vi "setIDtoVD.vi"(0 "Interface in":T4, 5 "IDtoVD":T1={"gains"={"proportional gain"=0.0, "integral gain"=0.0}, "output range"={"output high (Inf)"=inf, "output low (-Inf)"=-inf}, "PI_state"=enum."idle", "reset"=FALSE, "manual"=0.0} {"gains"."proportional gain" step=0.125}, 11 "error in":errorcluster) -> (4 "Interface out":T4, 15 "error out":errorcluster)   [LabVIEW 2017, in "AFE_interface.lvlib"]
uses:
  AFE_interface.lvlib
  InterfaceRef.ctl
  <instrlib>/_niInstr/Instruction Framework/v1/Host/Instruction Target/niInstr Instruction Target v1 Host.lvclass
  <instrlib>/_niInstr/Instruction Framework/v1/Host/Instruction Framework Context/niInstr Instruction Framework Context v1 Host.lvclass
  AFE/PI_Settings.ctl
  <vilib>/rvi/Analysis/control/PID/Typedef/niFpgaPID_PIGains.ctl
  <vilib>/rvi/Analysis/control/PID/Typedef/niFpgaPID_OutputRange.ctl
  <vilib>/NI/JSON Support for LabVIEW/JSON Data Classes/JSON Object/JSON Object.lvclass
  C:/Program Files (x86)/National Instruments/LabVIEW 2017/vi.lib/NI/JSON Support for LabVIEW/JSON Data Classes/JSON Datatype/JSON Null.lvclass
  <vilib>/NI/JSON Support for LabVIEW/JSON Data Classes/JSON Object/New JSON Object (Empty).vi
  <vilib>/NI/JSON Support for LabVIEW/JSON Data Classes/JSON Helper/Parsing/Parse Value.vi
  <vilib>/NI/JSON Support for LabVIEW/JSON Data Classes/JSON Object/Insert Key Value Pair.vi
  <vilib>/NI/JSON Support for LabVIEW/JSON Data Classes/JSON Object/Insert Key Value Pair (Single).vi
  <vilib>/NI/JSON Support for LabVIEW/JSON Data Classes/JSON Helper/To File (Path).vi
  <vilib>/NI/JSON Support for LabVIEW/JSON Data Classes/JSON Datatype/JSON Null.lvclass
  <vilib>/NI/JSON Support for LabVIEW/JSON Data Classes/JSON Object/Set Object Parameters XNode/Set Object Parameters.xnode
  <vilib>/NI/JSON Support for LabVIEW/JSON Data Classes/JSON Helper/JSON Helper.lvclass
  C:/Program Files (x86)/National Instruments/LabVIEW 2017/vi.lib/NI/JSON Support for LabVIEW/JSON Data Classes/JSON Structured Type/JSON Structure.lvclass
  AFE/ActiveFrontEnd.lvlib
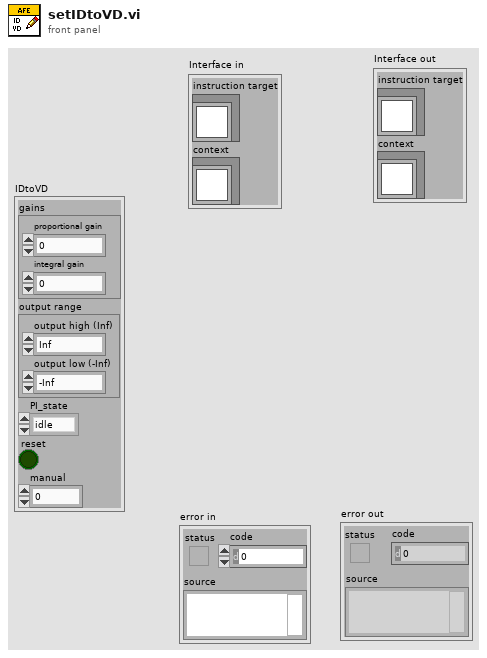
[diagram p1: front panel]
types:
  T1 = typedef "ActiveFrontEnd.lvlib/PI_Settings.ctl" = cluster{"gains":T2, "output range":T3, "PI_state":enum8{"idle", "normal", "manual", "perturbance"}, "reset":bool, "manual":sgl}
  T2 = typedef "niFpgaPID_PIGains.ctl" = cluster{"proportional gain":sgl, "integral gain":sgl}
  T3 = typedef "niFpgaPID_OutputRange.ctl" = cluster{"output high (Inf)":sgl, "output low (-Inf)":sgl}
  T4 = typedef "AFE_interface.lvlib/InterfaceRef.ctl" = cluster{"instruction target":refnum<class "niInstr Instruction Target v1 Host.lvclass">, "context":refnum<class "niInstr Instruction Framework Context v1 Host.lvclass">}
  T5 = enum16{"open", "replace", "create", "open or create", "replace or create", "replace or create with confirmation"}
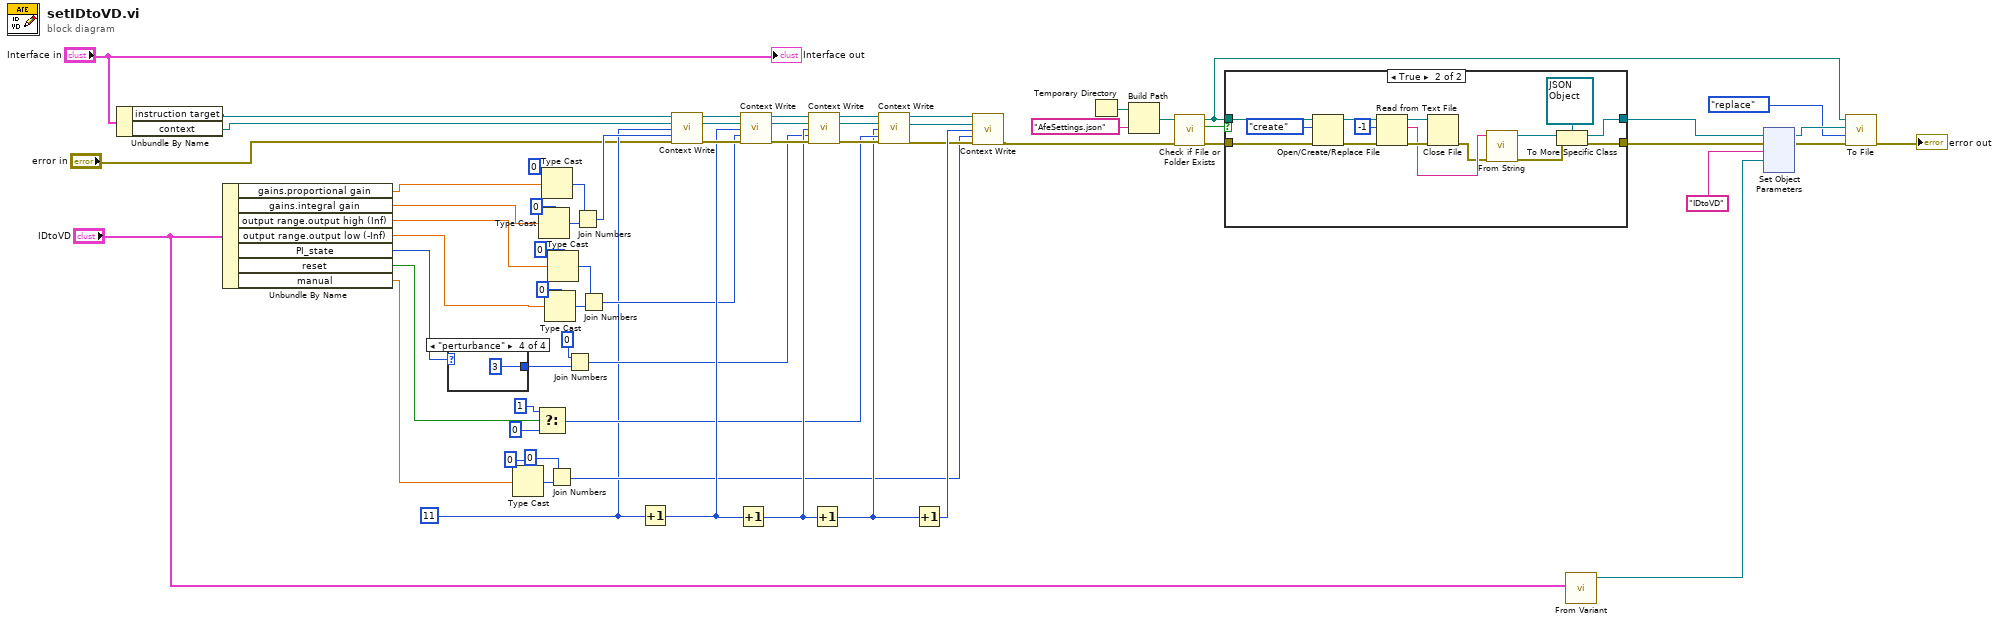
[diagram p0: block diagram]
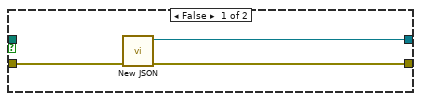
[diagram p2: hidden frame]
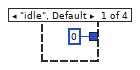
[diagram p3: hidden frame]
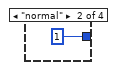
[diagram p4: hidden frame]
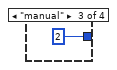
[diagram p5: hidden frame]
diagram:
  w18 = 11 ("x")
  n1 = Unbundle By Name("Interface in") -> ("instruction target"=w20:refnum<class "niInstr Instruction Target v1 Host.lvclass">, "context"=w19:refnum<class "niInstr Instruction Framework Context v1 Host.lvclass">)
  n2 = Unbundle By Name("IDtoVD") -> ("gains.proportional gain"=w49:sgl, "gains.integral gain"=w48:sgl, "output range.output high (Inf)"=w42:sgl, "output range.output low (-Inf)"=w41:sgl, "PI_state"=w23:enum8{"idle", "normal", "manual", "perturbance"}, "reset"=w40:bool, "manual"=w26:sgl)
  n3 = case shown="\"perturbance\"" w23 {
    tunnel: [u32 0 u32 1 u32 2 u32 3] -> w22
    frame "idle", Default {
    }
    frame "normal" {
    }
    frame "manual" {
    }
    frame "perturbance" {
    }
  }
  n4 = Type Cast(type=u32 0, x=w26) -> (*(type *) &x=w28:u32)
  n5 = Select(t=u64 1 ("data"), s=w40, f=u64 0) -> (s? t:f=w35:u64)
  n6 = Type Cast(type=u32 0, x=w48) -> (*(type *) &x=w50:u32)
  n7 = Type Cast(type=u32 0, x=w49) -> (*(type *) &x=w53:u32)
  n8 = Type Cast(type=u32 0, x=w41) -> (*(type *) &x=w46:u32)
  n9 = Join Numbers(hi=u32 0, lo=w28) -> ((hi.lo)=w24:u64)
  n10 = Type Cast(type=u32 0, x=w42) -> (*(type *) &x=w43:u32)
  n11 = Join Numbers(hi=u32 0, lo=w22) -> ((hi.lo)=w38:u64)
  n12 = Join Numbers(hi=w53, lo=w50) -> ((hi.lo)=w47:u64)
  n13 = Join Numbers(hi=w43, lo=w46) -> ((hi.lo)=w39:u64)
  n14 = Increment(x=w18) -> (x+1=w55:i32)
  n15 = call <instrlib>:"Context Write.vi"("instruction target in"=w20, "context in"=w19, "address"=w18, "data"=w47, "error in"="error in") -> ("instruction target out"=w64:refnum<class "niInstr Instruction Target v1 Host.lvclass">, "context out"=w61:refnum<class "niInstr Instruction Framework Context v1 Host.lvclass">, "error out"=w58:errorcluster)  [unwired: 8 in]
  n16 = Increment(x=w55) -> (x+1=w54:i32)
  n17 = call <instrlib>:"Context Write.vi"("instruction target in"=w64, "context in"=w61, "address"=w55, "data"=w39, "error in"=w58) -> ("instruction target out"=w63:refnum<class "niInstr Instruction Target v1 Host.lvclass">, "context out"=w60:refnum<class "niInstr Instruction Framework Context v1 Host.lvclass">, "error out"=w57:errorcluster)  [unwired: 8 in]
  n18 = call <instrlib>:"Context Write.vi"("instruction target in"=w63, "context in"=w60, "address"=w54, "data"=w38, "error in"=w57) -> ("instruction target out"=w62:refnum<class "niInstr Instruction Target v1 Host.lvclass">, "context out"=w59:refnum<class "niInstr Instruction Framework Context v1 Host.lvclass">, "error out"=w56:errorcluster)  [unwired: 8 in]
  n19 = Increment(x=w54) -> (x+1=w33:i32)
  n20 = call <instrlib>:"Context Write.vi"("instruction target in"=w62, "context in"=w59, "address"=w33, "data"=w35, "error in"=w56) -> ("instruction target out"=w31:refnum<class "niInstr Instruction Target v1 Host.lvclass">, "context out"=w30:refnum<class "niInstr Instruction Framework Context v1 Host.lvclass">, "error out"=w29:errorcluster)  [unwired: 8 in]
  n21 = Increment(x=w33) -> (x+1=w32:i32)
  n22 = call <instrlib>:"Context Write.vi"("instruction target in"=w31, "context in"=w30, "address"=w32, "data"=w24, "error in"=w29) -> ("error out"=w3:errorcluster)  [unwired: 8 in, 2 out]
  n23 = Temporary Directory() -> (w16:path)
  n24 = Build Path(base path=w16, name or relative path="AfeSettings.json") -> (appended path=w13:path)
  n25 = call <vilib>:"Check if File or Folder Exists.vi"("error in (no error)"=w3, "path"=w13) -> ("error out"=w14:errorcluster, "file or folder exists?"=w12:bool, "dup path"=w5:path)  [unwired: 7 in]
  n26 = case shown="True" w12 {
    tunnel: w14 -> [w71 w80]
    tunnel: w5 -> [_ w79]
    tunnel: [w70 w74] -> w11
    tunnel: [w69 w73] -> w9
    frame False {
      n27 = call-poly <vilib>:"New JSON.vi"("error in (no error)"=w71) -> ("error out"=w69:errorcluster, "JSON Object out"=w70:refnum<class "JSON Object.lvclass">)  [unwired: 9 in]
    }
    frame True {
      n28 = Open/Create/Replace File(file path (use dialog)=w79, error in=w80, operation (0:open)=T5."create") -> (refnum out=w85:refnum<file>, error out=w86:errorcluster)  [unwired: 3 in, 1 out]
      n29 = Read from Text File(file (use dialog)=w85, count=-1, error in=w86) -> (refnum out=w77:refnum<file>, text=w76:string, error out=w78:errorcluster)  [unwired: 1 in, 1 out]
      n30 = Close File(refnum=w77, error in=w78) -> (error out=w75:errorcluster)  [unwired: 1 out]
      n31 = call <vilib>:"From String.vi"("error in (no error)"=w75, "JSON String"=w76) -> ("error out"=w83:errorcluster, "JSON out"=w82:refnum<class "JSON Null.lvclass">)  [unwired: 8 in]
      n32 = To More Specific Class(target class=refnum<class "JSON Object.lvclass"> refnum ("JSON Object In"), reference=w82, error in=w83) -> (specific class reference=w74:refnum<class "JSON Object.lvclass">, error out=w73:errorcluster)
    }
  }
  n33 = call <vilib>:"From Variant.vi"("Variant"="IDtoVD") -> ("JSON out"=w10:refnum<class "JSON Null.lvclass">)  [unwired: 9 in, 1 out]
  n34 = xnode "Set Object Parameters"("key"="IDtoVD", "parameter"=w10, "JSON Object In"=w11, "error in"=w9) -> ("JSON Object Out"=w6:refnum<class "JSON Object.lvclass">, "error out"=w7:errorcluster)  [unwired: 1 out]
  n35 = call-poly <vilib>:"To File.vi"("error in (no error)"=w7, "operation (0:open)"=T5."replace", "JSON Datatype in"=w6, "file path"=w5) -> ("error out"=→"error out":errorcluster)  [unwired: 7 in]
  "Interface out" <- "Interface in"
